vi "Drive.vi"() -> ()   [LabVIEW 2019]
uses:
  <vilib>/Rock Robotics/SystemInterfaces/AI/FPGA_AIChannel.ctl
  Drive Global.vi
panel:
  out "Back Right":dbl
  out "Back Left":dbl
  out "Front Right":dbl
  out "Front Left":dbl
  in  "Pot values":T1
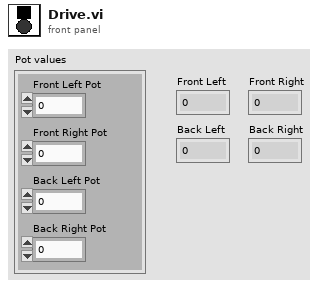
[diagram p1: front panel]
types:
  T1 = cluster{"Front Left Pot":dbl, "Front Right Pot":dbl, "Back Left Pot":dbl, "Back Right Pot":dbl}
  T2 = typedef "FPGA_AIChannel.ctl" = enum8{"AI 0", "AI 1", "AI 2", "AI 3", "AI MXP 0", "AI MXP 1", "AI MXP 2", "AI MXP 3", "Invalid"}
  T3 = typedef "WPI_MotorControlDeviceRef.ctl" = cluster{"DeviceStatus":errorcluster, "Type":T4, "PWM":cluster{"PWM Channel":T5, "DeadBand":T6}, "CAN":cluster{"Device Number":u8, "SetOutput VI Ref":variant, "GetOutput VI Ref":variant, "Enable VI Ref":variant, "Disable VI Ref":variant, "Data":variant}, "Invert":bool, "DIO PWM":cluster{"PWM \"Enable\" Channel":T5, "DIOChannel":T7, "PWM Rate":dbl}}
  T4 = typedef "WPI_MotorControlType.ctl" = enum16{"PWM", "CAN", "DIO PWM"}
  T5 = typedef "FPGA_DIOPWMChannel.ctl" = enum8{"PWM 0", "PWM 1", "PWM 2", "PWM 3", "PWM 4", "PWM 5", "PWM 6", "PWM 7", "PWM 8", "PWM 9", "PWM MXP 0", "PWM MXP 1", "PWM MXP 2", "PWM MXP 3", "PWM MXP 4", "PWM MXP 5", "PWM MXP 6", "PWM MXP 7", "PWM MXP 8", "PWM MXP 9", "Invalid"}
  T6 = typedef "WPI_PWMDeadband.ctl" = cluster{"Name":string, "maxPositivePwm":i32, "minPositivePwm":i32, "centerPwm":i32, "maxNegativePwm":i32, "minNegativePwm":i32, "angularRange":u16}
  T7 = typedef "FPGA_DIOChannel.ctl" = enum8{"DIO 0", "DIO 1", "DIO 2", "DIO 3", "DIO 4", "DIO 5", "DIO 6", "DIO 7", "DIO 8", "DIO 9", "DIO MXP 0", "DIO MXP 1", "DIO MXP 2", "DIO MXP 3", "DIO MXP 4", "DIO MXP 5", "DIO MXP 6", "DIO MXP 7", "DIO MXP 8", "DIO MXP 9", "DIO MXP 10", "DIO MXP 11", "DIO MXP 12", "DIO MXP 13", "DIO MXP 14", "DIO MXP 15", "SPI Port CS1", "SPI Port CS2", "SPI Port CS3", "SPI Port MISO", "SPI Port MOSI", "Invalid"}
  T8 = typedef "WPI_PotentiometerDevRef.ctl" = cluster{"DevStatus":errorcluster, "Analog Channel":T2, "Invert Output":bool}
  T9 = cluster{"Y Command":dbl, "X Command":dbl, "Z Command":dbl}
  T10 = cluster{"Front Left Offset":dbl, "Front Right Offset":dbl, "Back Left Offset":dbl, "Back Right Offset":dbl}
  T11 = cluster{"Z":dbl, "Y":dbl, "X":dbl, "Rot Point X":dbl, "Rot Point Y":dbl, "Width / 2":dbl, "Z Max":dbl, "Length / 2":dbl, "[8]":dbl}
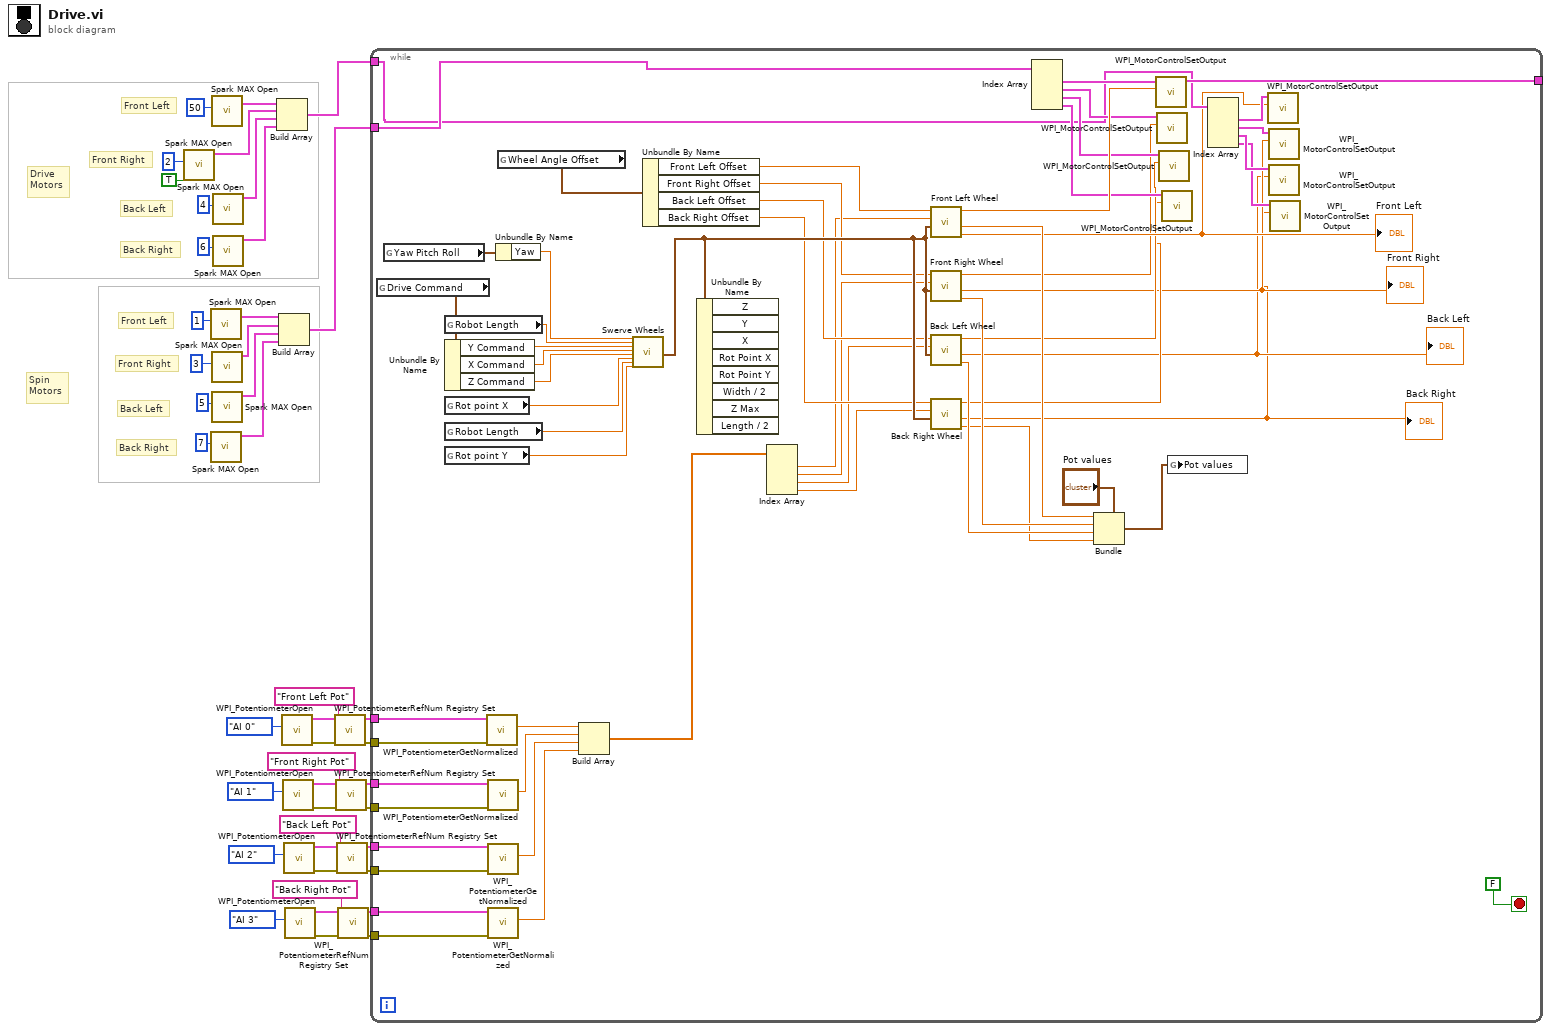
[diagram p0: block diagram]
diagram:
  # "Spin\nMotors"
  # "Drive \nMotors"
  # "Back Right"
  # "Back Left"
  # "Front Right"
  # "Front Left"
  # "Back Right"
  # "Back Left"
  # "Front Right"
  # "Front Left"
  n1 = call <vilib>:"Spark MAX Open.vi"("Invert"=TRUE, "Device Number"=u8 2) -> ("MotorControlDeviceRef"=w38:T3)  [unwired: 8 in, 1 out]
  n2 = call <vilib>:"Spark MAX Open.vi"("Device Number"=u8 1) -> ("MotorControlDeviceRef"=w31:T3)  [unwired: 9 in, 1 out]
  n3 = call <vilib>:"Spark MAX Open.vi"("Device Number"=u8 7) -> ("MotorControlDeviceRef"=w34:T3)  [unwired: 9 in, 1 out]
  n4 = call <vilib>:"Spark MAX Open.vi"("Device Number"=u8 50) -> ("MotorControlDeviceRef"=w39:T3)  [unwired: 9 in, 1 out]
  n5 = call <vilib>:"Spark MAX Open.vi"("Device Number"=u8 3) -> ("MotorControlDeviceRef"=w32:T3)  [unwired: 9 in, 1 out]
  n6 = call <vilib>:"Spark MAX Open.vi"("Device Number"=u8 5) -> ("MotorControlDeviceRef"=w33:T3)  [unwired: 9 in, 1 out]
  n7 = call <vilib>:"Spark MAX Open.vi"("Device Number"=u8 4) -> ("MotorControlDeviceRef"=w37:T3)  [unwired: 9 in, 1 out]
  n8 = call <vilib>:"Spark MAX Open.vi"("Device Number"=u8 6) -> ("MotorControlDeviceRef"=w36:T3)  [unwired: 9 in, 1 out]
  n9 = Build Array(w39, w38, w37, w36) -> (w35:T3[])
  n10 = Build Array(w31, w32, w33, w34) -> (w29:T3[])
  n11 = call <vilib>:"WPI_PotentiometerOpen.vi"("Analog Channel"=FPGA_AIChannel."AI 0") -> ("error out"=w27:errorcluster, "PotDevRef"=w26:T8)  [unwired: 9 in]
  n12 = call <vilib>:"WPI_PotentiometerOpen.vi"("Analog Channel"=FPGA_AIChannel."AI 1") -> ("error out"=w22:errorcluster, "PotDevRef"=w23:T8)  [unwired: 9 in]
  n13 = call <vilib>:"WPI_PotentiometerOpen.vi"("Analog Channel"=FPGA_AIChannel."AI 2") -> ("error out"=w14:errorcluster, "PotDevRef"=w15:T8)  [unwired: 9 in]
  n14 = call <vilib>:"WPI_PotentiometerOpen.vi"("Analog Channel"=FPGA_AIChannel."AI 3") -> ("error out"=w19:errorcluster, "PotDevRef"=w18:T8)  [unwired: 9 in]
  n15 = call <vilib>:"WPI_PotentiometerRefNum Registry Set.vi"("error in (no error)"=w27, "refnum name"="Front Left Pot", "PotDevRef"=w26) -> ("error out"=w11:errorcluster, "PotDevRef"=w12:T8)  [unwired: 7 in]
  n16 = call <vilib>:"WPI_PotentiometerRefNum Registry Set.vi"("error in (no error)"=w22, "refnum name"="Front Right Pot", "PotDevRef"=w23) -> ("error out"=w9:errorcluster, "PotDevRef"=w10:T8)  [unwired: 7 in]
  n17 = call <vilib>:"WPI_PotentiometerRefNum Registry Set.vi"("error in (no error)"=w14, "refnum name"="Back Left Pot", "PotDevRef"=w15) -> ("error out"=w7:errorcluster, "PotDevRef"=w8:T8)  [unwired: 7 in]
  n18 = call <vilib>:"WPI_PotentiometerRefNum Registry Set.vi"("error in (no error)"=w19, "refnum name"="Back Right Pot", "PotDevRef"=w18) -> ("error out"=w5:errorcluster, "PotDevRef"=w6:T8)  [unwired: 7 in]
  n19 = while {
    tunnel: w35 -> [w55]
    tunnel: w29 -> [w62]
    tunnel: w12 -> [w81]
    tunnel: w11 -> [w80]
    tunnel: w10 -> [w79]
    tunnel: w9 -> [w78]
    tunnel: w8 -> [w77]
    tunnel: w7 -> [w76]
    tunnel: w6 -> [w75]
    tunnel: w5 -> [w74]
    tunnel: [w66] -> _
    stop <- FALSE stop-if-true
    n20 = global read "Drive Global.vi" "Drive Command"() -> (w91:T9)
    n21 = global read "Drive Global.vi" "Yaw Pitch Roll"() -> (w101:cluster{"Yaw":dbl, "Pitch":dbl, "Roll":dbl})
    n22 = global read "Drive Global.vi" "Robot Length"() -> (w86:dbl)
    n23 = Unbundle By Name(w91) -> ("Y Command"=w90:dbl, "X Command"=w89:dbl, "Z Command"=w88:dbl)
    n24 = global read "Drive Global.vi" "Rot point X"() -> (w99:dbl)
    n25 = global read "Drive Global.vi" "Robot Length"() -> (w87:dbl)
    n26 = global read "Drive Global.vi" "Rot point Y"() -> (w98:dbl)
    n27 = call <vilib>:"WPI_PotentiometerGetNormalized.vi"("error in"=w80, "PotDevRef"=w81) -> ("Normalized Value"=w85:dbl)  [unwired: 7 in, 2 out]
    n28 = call <vilib>:"WPI_PotentiometerGetNormalized.vi"("error in"=w78, "PotDevRef"=w79) -> ("Normalized Value"=w84:dbl)  [unwired: 7 in, 2 out]
    n29 = call <vilib>:"WPI_PotentiometerGetNormalized.vi"("error in"=w76, "PotDevRef"=w77) -> ("Normalized Value"=w83:dbl)  [unwired: 7 in, 2 out]
    n30 = call <vilib>:"WPI_PotentiometerGetNormalized.vi"("error in"=w74, "PotDevRef"=w75) -> ("Normalized Value"=w82:dbl)  [unwired: 7 in, 2 out]
    n31 = Unbundle By Name(w101) -> ("Yaw"=w100:dbl)
    n32 = global read "Drive Global.vi" "Wheel Angle Offset"() -> (w96:T10)
    n33 = Build Array(w85, w84, w83, w82) -> (w73:dbl[])
    n34 = call "Swerve Wheels.vi"("Yaw"=w100, "Robot Width"=w86, "Y Command"=w90, "X Command"=w89, "Z Command"=w88, "Rot. Point X"=w99, "Robot  Length"=w87, "Rot. Point Y"=w98) -> ("output cluster"=w97:T11)  [unwired: 19 in]
    n35 = Unbundle By Name(w96) -> ("Front Left Offset"=w95:dbl, "Front Right Offset"=w94:dbl, "Back Left Offset"=w93:dbl, "Back Right Offset"=w92:dbl)
    n36 = Unbundle By Name(w97) -> ()  [unwired: 8 out]
    n37 = Index Array(array=w73) -> (element #1=w69:dbl, element #2=w70:dbl, element #3=w71:dbl, element #4=w72:dbl)  [unwired: 4 in]
    n38 = call "Front Left Wheel.vi"("output cluster 2"=w97, "Pot Val in"=w69, "Wheel Angle Offset"=w95) -> ("Drive Speed"=w52:dbl, "Wheel Angle"=w61:dbl, "Wheel Speed"=w67:dbl)  [unwired: 6 in]
    "Front Left" <- w52
    n39 = call "Front Right Wheel.vi"("output cluster 2"=w97, "Pot Val in"=w70, "Wheel Angle Offset"=w94) -> ("Wheel Angle"=w59:dbl, "Drive Speed"=w46:dbl, "Wheel Speed"=w49:dbl)  [unwired: 6 in]
    "Front Right" <- w46
    n40 = call "Back Left Wheel.vi"("output cluster 2"=w97, "Pot Val in"=w71, "Wheel Angle Offset"=w93) -> ("Wheel Angle"=w60:dbl, "Drive Speed"=w45:dbl, "Wheel Speed"=w48:dbl)  [unwired: 5 in]
    "Back Left" <- w45
    n41 = call "Back Right Wheel.vi"("output cluster 2"=w97, "Pot Val in"=w72, "Wheel Angle Offset"=w92) -> ("Wheel Angle"=w58:dbl, "Drive Speed"=w44:dbl, "Wheel Speed"=w47:dbl)  [unwired: 6 in]
    "Back Right" <- w44
    n42 = Index Array(array=w62) -> (element #1=w68:T3, element #2=w65:T3, element #3=w64:T3, element #4=w63:T3)  [unwired: 4 in]
    n43 = Bundle(cluster="Pot values", "Front Left Pot"=w61, "Front Right Pot"=w59, "Back Left Pot"=w60, "Back Right Pot"=w58) -> (w56:T1)
    n44 = call <vilib>:"WPI_MotorControlSetOutput.vi"("Output"=w67, "MotorControlDevRef"=w68) -> ("MotorControlDevRef"=w66:T3)  [unwired: 7 in, 2 out]
    n45 = call <vilib>:"WPI_MotorControlSetOutput.vi"("Output"=w49, "MotorControlDevRef"=w65) -> ()  [unwired: 7 in, 3 out]
    n46 = call <vilib>:"WPI_MotorControlSetOutput.vi"("Output"=w48, "MotorControlDevRef"=w64) -> ()  [unwired: 7 in, 3 out]
    n47 = call <vilib>:"WPI_MotorControlSetOutput.vi"("Output"=w47, "MotorControlDevRef"=w63) -> ()  [unwired: 7 in, 3 out]
    n48 = global write "Drive Global.vi" "Pot values"(w56) -> ()
    n49 = Index Array(array=w55) -> (element #1=w54:T3, element #2=w53:T3, element #3=w51:T3, element #4=w50:T3)  [unwired: 4 in]
    n50 = call <vilib>:"WPI_MotorControlSetOutput.vi"("Output"=w52, "MotorControlDevRef"=w54) -> ()  [unwired: 7 in, 3 out]
    n51 = call <vilib>:"WPI_MotorControlSetOutput.vi"("Output"=w46, "MotorControlDevRef"=w53) -> ()  [unwired: 7 in, 3 out]
    n52 = call <vilib>:"WPI_MotorControlSetOutput.vi"("Output"=w45, "MotorControlDevRef"=w51) -> ()  [unwired: 7 in, 3 out]
    n53 = call <vilib>:"WPI_MotorControlSetOutput.vi"("Output"=w44, "MotorControlDevRef"=w50) -> ()  [unwired: 7 in, 3 out]
  }
